vi "get valid output path.vi"(8 "error in (no error)":errorcluster, 11 "TDMS datalogger configuration in":refnum<class "TDMS datalogger configuration.lvclass">) -> (0 "error out":errorcluster, 2 "Path":path, 3 "TDMS datalogger configuration out":refnum<class "TDMS datalogger configuration.lvclass">)   [LabVIEW 2013, in "TDMS datalogger configuration.lvclass"]
uses:
  TDMS datalogger configuration.lvclass
  TDMS datalogger configuration.lvclass/TDMS datalogger configuration.ctl
  <vilib>/NI/Configuration Framework/serializable configuration/NISE_CEF_serializable configuration.lvclass/NISE_CEF_serializable configuration.ctl
  Read Path.vi
  Read log name.vi
  <vilib>/NI/Configuration Framework/serializable configuration/Read UID.vi
  <vilib>/Utility/LVClass/Get LV Class Name.vi
  <vilib>/NI/Configuration Framework/error generator/NISE_error generator.vi
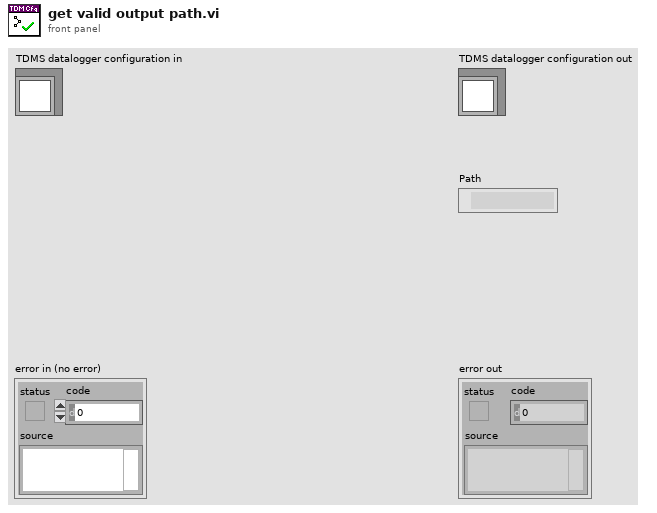
[diagram p1: front panel]
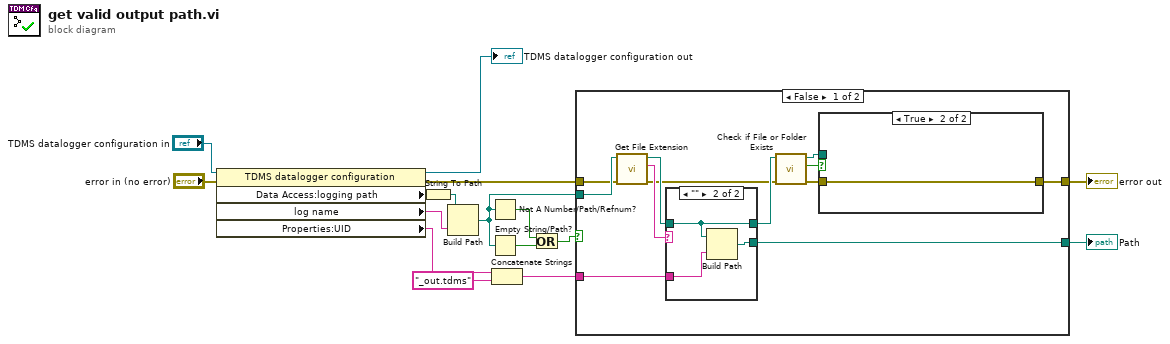
[diagram p0: block diagram]
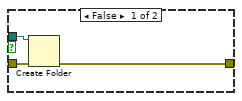
[diagram p2: hidden frame]
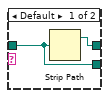
[diagram p3: hidden frame]
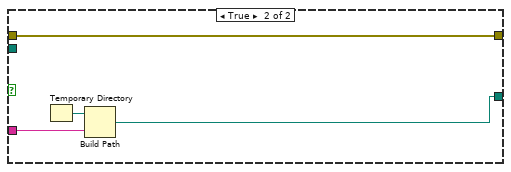
[diagram p4: hidden frame]
diagram:
  n1 = property class="TDMS datalogger configuration"(reference="TDMS datalogger configuration in", error in="error in (no error)") -> (reference out=→"TDMS datalogger configuration out":refnum<class "TDMS datalogger configuration.lvclass">, error out=w13:errorcluster, "Data Access:logging path"=w4:string, "log name"=w2:string, "Properties:UID"=w11:string)
  n2 = String To Path(string=w4) -> (path=w3:path)
  n3 = Build Path(base path=w3, name or relative path=w2) -> (appended path=w1:path)
  n4 = Not A Number/Path/Refnum?(number/path/refnum=w1) -> (NaN/Path/Refnum?=w15:bool)
  n5 = Empty String/Path?(string/path=w1) -> (empty?=w16:bool)
  n6 = Concatenate Strings(w11, "_out.tdms" ("string")) -> (w10:string)
  n7 = Or(x=w15, y=w16) -> (x .or. y?=w14:bool)
  n8 = case shown="False" w14 {
    tunnel: [w23 w40] -> w9
    tunnel: w1 -> [w28 _]
    tunnel: w13 -> [w27 w38]
    tunnel: w10 -> [w24 w39]
    tunnel: [w19 w38] -> w8
    frame False {
      n9 = call <vilib>:"Get File Extension.vi"("error in (no error)"=w27, "file"=w28) -> ("error out"=w21:errorcluster, "lowercase file extension"=w25:string, "dup file"=w26:path)  [unwired: 6 in, 1 out]
      n10 = case shown="\"\"" w25 {
        tunnel: w26 -> [w34 w35]
        tunnel: w24 -> [_ w37]
        tunnel: [w34 w36] -> w23
        tunnel: [w33 w35] -> w22
        frame Default {
          n11 = Strip Path(path=w34) -> (stripped path=w33:path)  [unwired: 1 out]
        }
        frame "" {
          n12 = Build Path(base path=w35, name or relative path=w37) -> (appended path=w36:path)
        }
      }
      n13 = call <vilib>:"Check if File or Folder Exists.vi"("error in (no error)"=w21, "path"=w22) -> ("error out"=w18:errorcluster, "file or folder exists?"=w20:bool, "dup path"=w17:path)  [unwired: 7 in]
      n14 = case shown="True" w20 {
        tunnel: [w29 w32] -> w19
        tunnel: w18 -> [w30 w32]
        tunnel: w17 -> [w31 _]
        frame False {
          n15 = Create Folder(path (use dialog)=w31, error in=w30) -> (error out=w29:errorcluster)  [unwired: 1 in, 2 out]
        }
        frame True {
        }
      }
    }
    frame True {
      n16 = Temporary Directory() -> (w41:path)
      n17 = Build Path(base path=w41, name or relative path=w39) -> (appended path=w40:path)
    }
  }
  "error out" <- w8
  "Path" <- w9
